vi "GMM.vi"(9 "cof":dbl[][](array[numeric])) -> (0 "错误输出":errorcluster, 1 "sigema":dbl[][](array[numeric]) format="%#_13g", 2 "mu":dbl[][](array[numeric]) format="%#_13g", 3 "pai":dbl[](array[numeric]) format="%#_13g")   [LabVIEW 2018]
panel:
  out "mu大小":dbl[](array[numeric])
  out "sigma大小":dbl[](array[numeric])
  out "errlog 4":dbl[][](array[numeric]) format="%#_13g"
  out "post 3":dbl[][](array[numeric]) format="%#_13g"
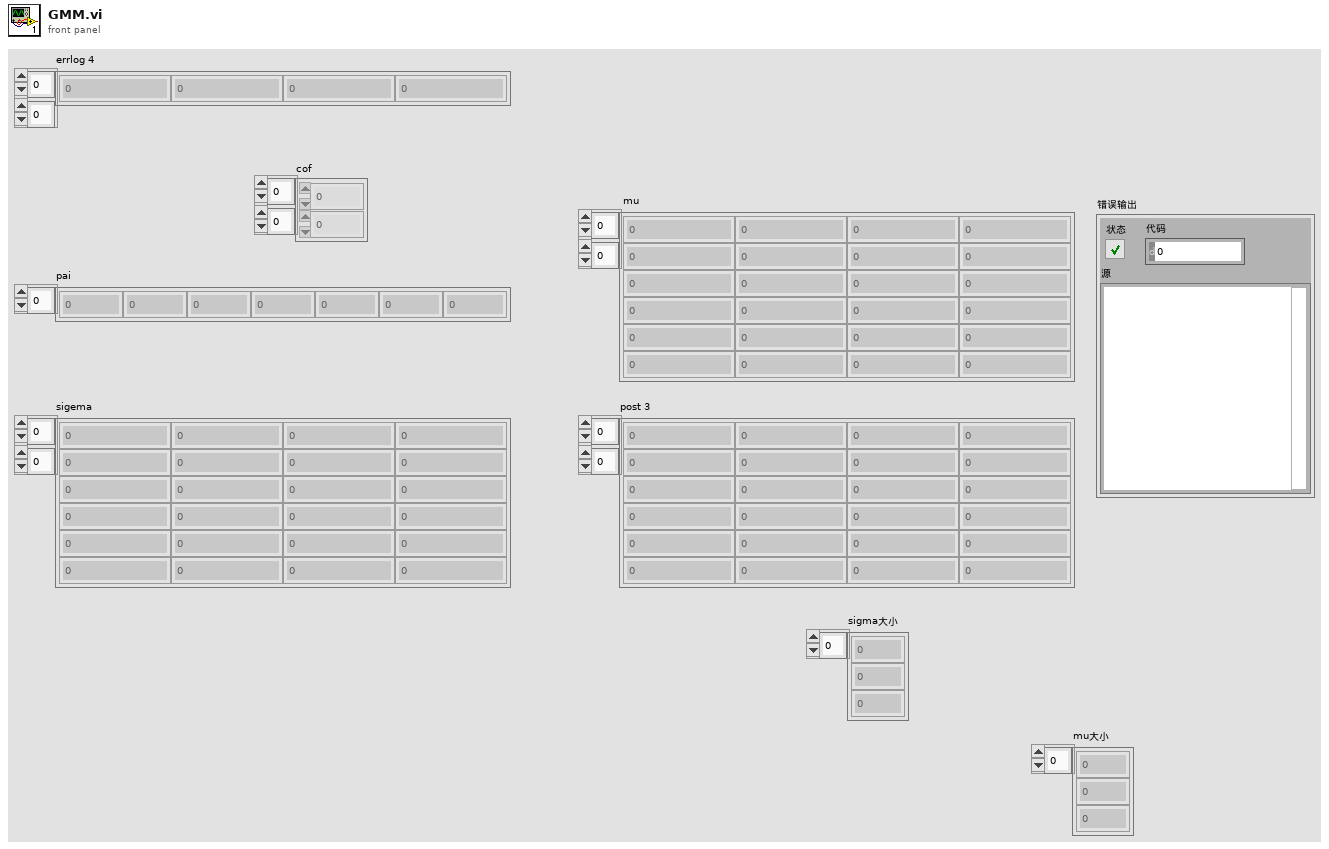
[diagram p1: front panel]
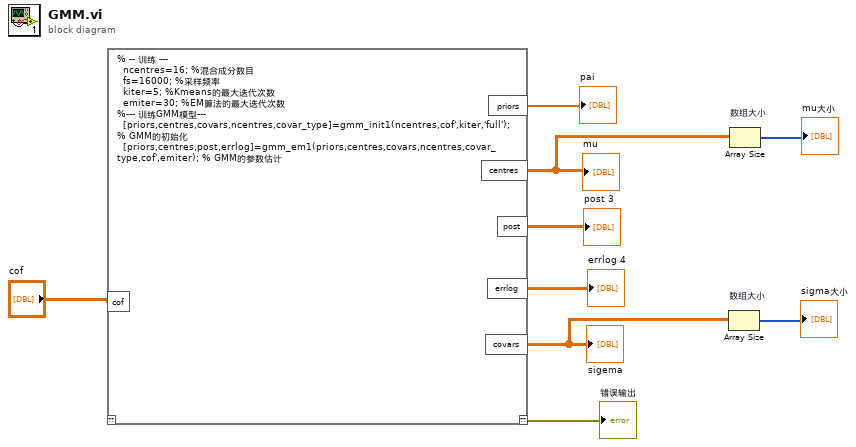
[diagram p0: block diagram]
diagram:
  n1 = script code="% -- 训练 ---\n  ncentres=16; %混合成分数目\n  fs=16000; %采样频率  \n  kiter=5; %Kmeans的最大迭代次数\n  emiter=30; %EM算法的最大迭代次数\n%--- 训练GMM模型---\n  [priors,centres,covars,ncentres,covar_type]=gmm_init1(ncentres,cof',kiter,'full'); % GMM的初始化\n  [priors,centres,post,errlog]=gmm_em1(priors,centres,covars,ncentres,covar_type,cof',emiter); % GMM的参数估计"("cof"="cof") -> ("??"=→"错误输出":errorcluster, "priors"=→"pai":dbl[], "centres"=w1:dbl[][], "post"=→"post 3":dbl[][], "errlog"=→"errlog 4":dbl[][], "covars"=w5:dbl[][])  [unwired: 1 in]
  "mu" <- w1
  "sigema" <- w5
  n2 = Array Size "数组大小"(array=w5) -> (size(s)=→"sigma大小":i32[])
  n3 = Array Size "数组大小"(array=w1) -> (size(s)=→"mu大小":i32[])
